vi "GetSetConfigClass.vi"(7 "Set (f)":bool, 11 "Ref in":refnum<class "Config.lvclass">) -> (3 "Ref out":refnum<class "Config.lvclass">)   [LabVIEW 2014, in "Config_class.lvlib" / "Config.lvclass"]
uses:
  Config.lvclass
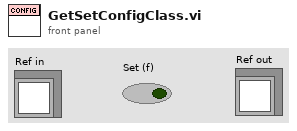
[diagram p1: front panel]
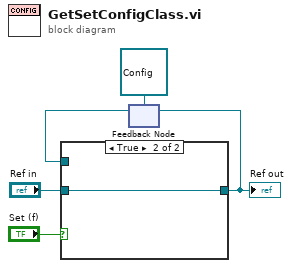
[diagram p0: block diagram]
diagram:
  n1 = feedback #1(refnum<class "Config.lvclass"> refnum ("Ref in")) -> (w2:refnum<class "Config.lvclass">)
  n2 = case shown="True" "Set (f)" {
    tunnel: "Ref in" -> [_ w7]
    tunnel: [w6 w7] -> w3
    tunnel: w2 -> [w6 _]
    frame False {
    }
    frame True {
    }
  }
  "Ref out" <- w3
  n3 = feedback-in #1(w3) -> ()
